vi "Terminate.vi"(8 "error in (no error)":errorcluster, 10 "Message in":refnum<class "TerminateMessage.lvclass">, 11 "DAQMH121119OrcaFlash in":refnum<class "DAQOrcaFlash.lvclass">) -> (0 "error out":errorcluster, 3 "DAQMH121119OrcaFlash out":refnum<class "DAQOrcaFlash.lvclass">)   [LabVIEW 2012, in "DAQOrcaFlash.lvclass"]
doc: "This member function is called when the statemachine in the run.vi receives an 'terminate' command. It closes the RabbitMQ connection. \n\nOverride this member function in your derived class to release all previously acquired resources (but don't forget to call the parent method). If your component has subcomponents, they count as resources, and you have to release them by calling their own terminate functions."
uses:
  DAQOrcaFlash.lvclass
  <vilib>/Distrio/Murmex/TerminateMessage/TerminateMessage.lvclass
  <vilib>/Distrio/Murmex/StopMessage/StopMessage.lvclass
  <vilib>/Distrio/Murmex/Murmex/Murmex.lvclass
panel:
  # "This method is called when the TERMINATE\ntrigger is sent. \n\nOverride this method when your component needs to\nrespond to this trigger. \n\nCall parent for proper implementation"
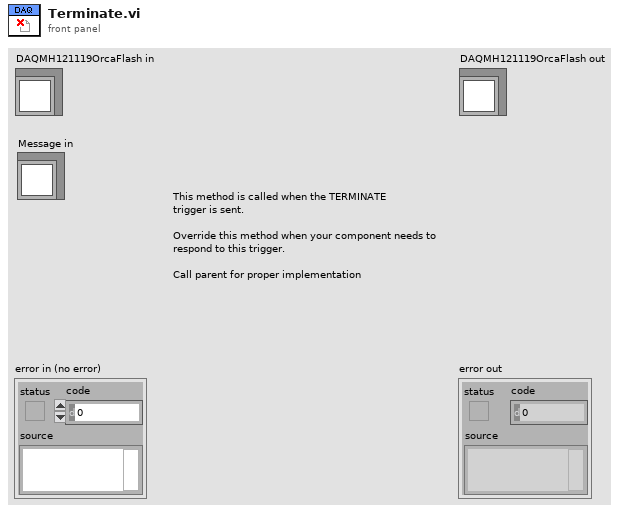
[diagram p1: front panel]
types:
  T1 = typedef "IMAQ Image.ctl" = refnum<image>
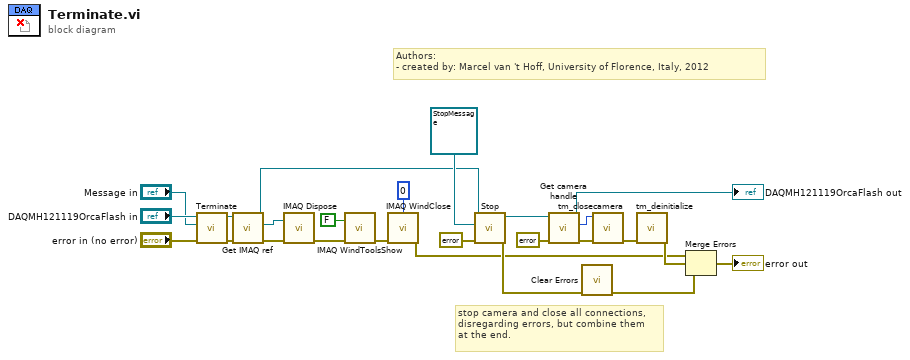
[diagram p0: block diagram]
diagram:
  # "stop camera and close all connections,\ndisregarding errors, but combine them\nat the end."
  # "Authors: \n- created by: Marcel van 't Hoff, University of Florence, Italy, 2012"
  n1 = call-parent "Terminate.vi"("error in (no error)"="error in (no error)", "Message in"="Message in", "Murmex in"="DAQMH121119OrcaFlash in") -> ("error out"=w8:errorcluster, "Murmex out"=w10:refnum<class "DAQOrcaFlash.lvclass">)  [unwired: 7 in]
  n2 = call "Get IMAQ ref.vi"("error in (no error)"=w8, "DAQMH121119OrcaFlash in"=w10) -> ("error out"=w5:errorcluster, "IMAQ reference"=w6:T1, "DAQMH121119OrcaFlash out"=w9:refnum<class "DAQOrcaFlash.lvclass">)  [unwired: 7 in]
  n3 = call "IMAQ Dispose"("Image"=w6, "error in (no error)"=w5) -> ("error out"=w4:errorcluster)  [unwired: 4 in]
  n4 = call "IMAQ WindToolsShow"("Hide/Show (Show)"=FALSE, "error in (no error)"=w4) -> ("error out"=w3:errorcluster)  [unwired: 3 in, 1 out]
  n5 = call "IMAQ WindClose"("Window Number (0...15)"=0, "error in (no error)"=w3) -> ("error out"=w1:errorcluster)  [unwired: 4 in]
  n6 = call-dynamic "Stop.vi"("error in (no error)"=errorcluster {"status"=FALSE, "code"=0, "source"=""}, "Message in"=refnum<class "StopMessage.lvclass"> refnum, "DAQMH121119OrcaFlash in"=w9) -> ("error out"=w13:errorcluster, "DAQMH121119OrcaFlash out"=w18:refnum<class "DAQOrcaFlash.lvclass">)  [unwired: 7 in]
  n7 = call "Get camera handle.vi"("error in (no error)"=errorcluster {"status"=FALSE, "code"=0, "source"=""}, "DAQMH121119OrcaFlash in"=w18) -> ("error out"=w19:errorcluster, "cam handle"=w20:u32, "DAQMH121119OrcaFlash out"=→"DAQMH121119OrcaFlash out":refnum<class "DAQOrcaFlash.lvclass">)  [unwired: 7 in]
  n8 = call <vilib>:"Clear Errors.vi"("error in (no error)"=w13) -> ("error out"=w11:errorcluster)  [unwired: 6 in]
  n9 = call <userlib>:"tm_closecamera.vi"("error in (no error)"=w19, "Handle in"=w20) -> ("error out"=w21:errorcluster)  [unwired: 9 in]
  n10 = call <userlib>:"tm_deinitialize.vi"("error in (no error)"=w21) -> ("error out"=w12:errorcluster)  [unwired: 10 in]
  n11 = Merge Errors(w1, w12, w11) -> (→"error out":errorcluster)
